vi "Read Analog Channel.vi"(8 "error in":errorcluster, 11 "analog channel in":refnum<class "Analog Channel.lvclass">) -> (0 "error out":errorcluster, 1 "default value":dbl, 2 "name":string, 3 "analog channel out":refnum<class "Analog Channel.lvclass">, 4 "index":i32)   [LabVIEW 2017, in "Scan Engine Scripting.lvlib" / "Analog Channel.lvclass"]
uses:
  Analog Channel.lvclass
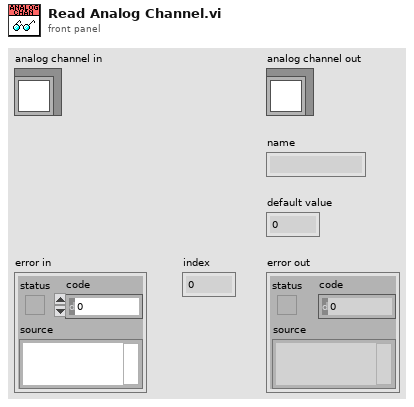
[diagram p1: front panel]
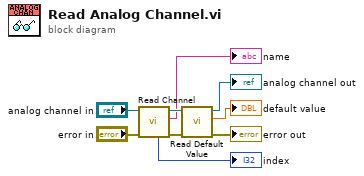
[diagram p0: block diagram]
diagram:
  n1 = call-dynamic "Read Channel.vi"("error in (no error)"="error in", "Channel in"="analog channel in") -> ("error out"=w6:errorcluster, "name"=→"name":string, "Channel out"=w7:refnum<class "Analog Channel.lvclass">, "index"=→"index":i32)  [unwired: 4 in, 2 out]
  n2 = call-dynamic "Read Default Value.vi"("error in"=w6, "analog channel in"=w7) -> ("error out"=→"error out":errorcluster, "default value"=→"default value":dbl, "analog channel out"=→"analog channel out":refnum<class "Analog Channel.lvclass">)  [unwired: 7 in]
